vi "JSON Value Probe.vi"(11 "JSON Value out":refnum<class "JSON Value.lvclass">) -> (2 "Value String":string, 3 "Boolean":bool)   [LabVIEW 2020, in "Library Commun.lvlib" / "JSON Value.lvclass"]
uses:
  JSON Value.lvclass
panel:
  out "JSON":string
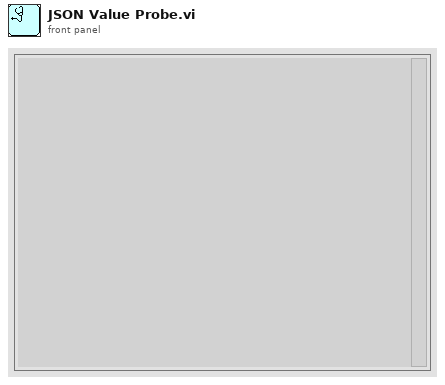
[diagram p1: front panel]
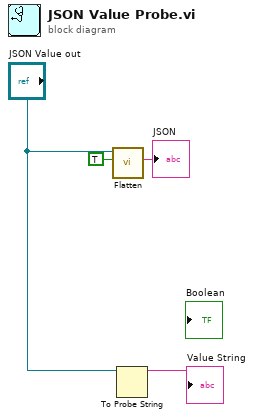
[diagram p0: block diagram]
diagram:
  n1 = call-dynamic "Flatten.vi"("Pretty Print?"=TRUE, "JSON Value in"="JSON Value out") -> ("<JSON>"=→"JSON":string)  [unwired: 8 in, 1 out]
  n2 = To Probe String(7:"JSON Value out") -> (3:→"Value String":string)  [unwired: 2 in, 1 out]
